vi "Initialize.vi"(2 "error in":errorcluster, 3 "VISA arduino in":refnum<visa-resource-name>) -> (0 "error out":errorcluster, 1 "VISA arduino out":refnum<visa-resource-name>)   [LabVIEW 2021]
uses:
  <vilib>/Instr/_visa.llb/VISA Configure Serial Port (Instr).vi
  <vilib>/Utility/error.llb/Error Cluster From Error Code.vi
  <vilib>/ErrorRing/Error Ring.xnode
panel:
  out "read buffer":string
  out "delay":u32
  out "max iterator":u8
  # "Private"
  # "Public"
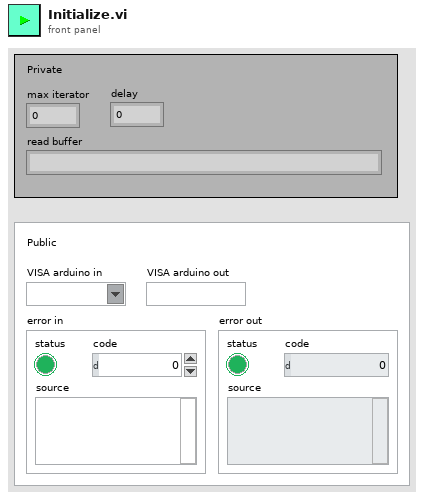
[diagram p1: front panel]
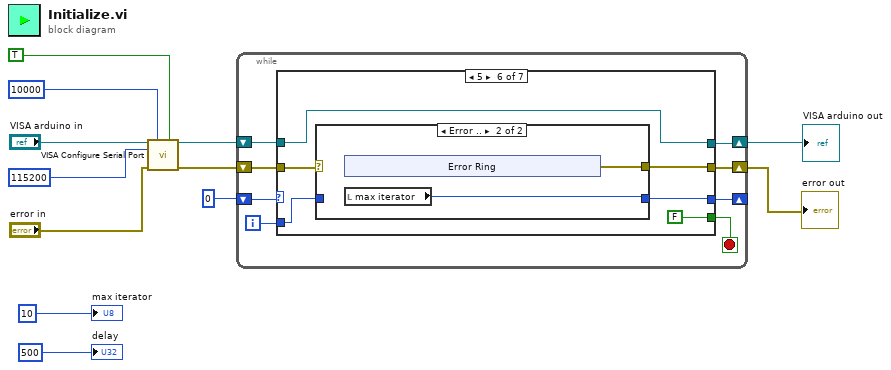
[diagram p0: block diagram]
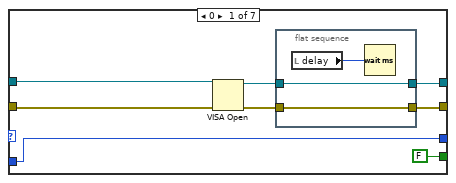
[diagram p2: hidden frame]
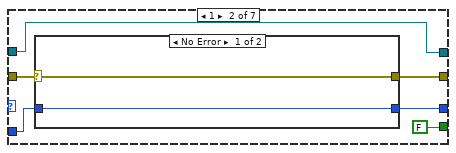
[diagram p3: hidden frame]
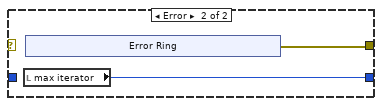
[diagram p4: hidden frame]
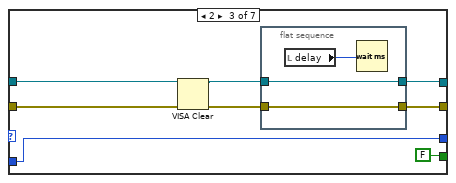
[diagram p5: hidden frame]
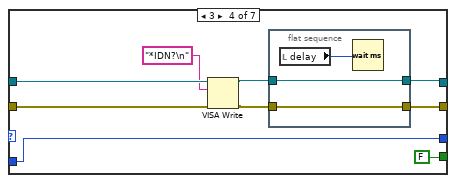
[diagram p6: hidden frame]
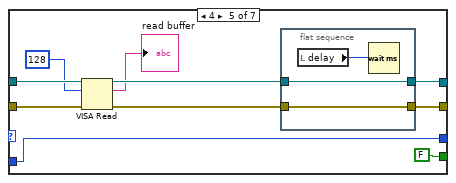
[diagram p7: hidden frame]
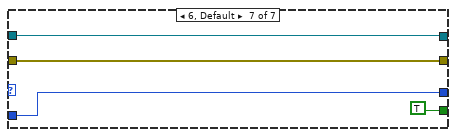
[diagram p9: hidden frame]
diagram:
  n1 = call-poly "VISA Configure Serial Port"("VISA resource name"="VISA arduino in", "timeout (10sec)"=u32 10000, "Enable Termination\nChar (T)"=TRUE ("Enable Termination\nChar (T)"), "baud rate (9600)"=u32 115200, "error in (no error)"="error in") -> ("VISA resource name out"=w9:refnum<visa-resource-name>, "error out"=w8:errorcluster)  [unwired: 9 in]
  n2 = while {
    shift-right: [w18] -> w1
    shift-left: w9 -> [w20]
    shift-right: [w17] -> w2
    shift-left: w8 -> [w19]
    shift-right: [w14] -> _
    shift-left: 0 -> [w16]
    i -> [w15]
    stop <- w13 stop-if-true
    n3 = case shown="5" w16 {
      tunnel: w20 -> [w28 w35 w54 w66 w79 w85 w101]
      tunnel: w19 -> [w27 w37 w53 w65 w78 w87 w100]
      tunnel: [w24 w35 w50 w59 w74 w85 w101] -> w18
      tunnel: [w22 w36 w48 w61 w72 w86 w100] -> w17
      tunnel: w15 -> [w26 w33 w52 w63 w76 w83 w99]
      tunnel: [w26 w34 w52 w63 w76 w84 w99] -> w14
      tunnel: [FALSE ("Enable Termination\nChar (T)") FALSE ("Enable Termination\nChar (T)") FALSE ("Enable Termination\nChar (T)") FALSE ("Enable Termination\nChar (T)") FALSE ("Enable Termination\nChar (T)") FALSE ("Enable Termination\nChar (T)") TRUE ("Enable Termination\nChar (T)")] -> w13
      frame 0 {
        n4 = VISA Open(error in (no error)=w27, VISA resource name=w28) -> (VISA resource name=w23:refnum<visa-resource-name>, error out=w21:errorcluster)  [unwired: 3 in]
        n5 = flat-sequence {
          tunnel: [w30] -> w24
          tunnel: w23 -> [w30]
          tunnel: [w29] -> w22
          tunnel: w21 -> [w29]
          frame #0 {
            n6 = local read "delay"() -> (w31:u32)
            n7 = Wait (ms)(milliseconds to wait=w31) -> ()  [unwired: 1 out]
          }
        }
      }
      frame 1 {
        n8 = case shown="No Error" w37 {
          selector: w37 -> [w39 _]
          tunnel: [w39 w40] -> w36
          tunnel: [w38 w41] -> w34
          tunnel: w33 -> [w38 _]
          frame No Error {
          }
          frame Error {
            n9 = local read "max iterator"() -> (w41:u8)
            n10 = xnode "Error Ring"() -> ("error out"=w40:errorcluster)
          }
        }
      }
      frame 2 {
        n11 = VISA Clear(VISA resource name=w54, error in (no error)=w53) -> (VISA resource name out=w49:refnum<visa-resource-name>, error out=w47:errorcluster)
        n12 = flat-sequence {
          tunnel: [w56] -> w50
          tunnel: w49 -> [w56]
          tunnel: [w55] -> w48
          tunnel: w47 -> [w55]
          frame #0 {
            n13 = local read "delay"() -> (w57:u32)
            n14 = Wait (ms)(milliseconds to wait=w57) -> ()  [unwired: 1 out]
          }
        }
      }
      frame 3 {
        n15 = VISA Write(VISA resource name=w66, write buffer="*IDN?\n", error in (no error)=w65) -> (VISA resource name out=w58:refnum<visa-resource-name>, error out=w60:errorcluster)  [unwired: 1 out]
        n16 = flat-sequence {
          tunnel: [w68] -> w61
          tunnel: w60 -> [w68]
          tunnel: [w67] -> w59
          tunnel: w58 -> [w67]
          frame #0 {
            n17 = local read "delay"() -> (w69:u32)
            n18 = Wait (ms)(milliseconds to wait=w69) -> ()  [unwired: 1 out]
          }
        }
      }
      frame 4 {
        n19 = VISA Read(VISA resource name=w79, byte count=u32 128, error in (no error)=w78) -> (VISA resource name out=w73:refnum<visa-resource-name>, read buffer=→"read buffer":string, error out=w71:errorcluster)  [unwired: 1 out]
        n20 = flat-sequence {
          tunnel: [w81] -> w74
          tunnel: w73 -> [w81]
          tunnel: [w80] -> w72
          tunnel: w71 -> [w80]
          frame #0 {
            n21 = local read "delay"() -> (w82:u32)
            n22 = Wait (ms)(milliseconds to wait=w82) -> ()  [unwired: 1 out]
          }
        }
      }
      frame 5 {
        n23 = case shown="Error .." w87 {
          selector: w87 -> [w90 _]
          tunnel: [w90 w92] -> w86
          tunnel: [w89 w91] -> w84
          tunnel: w83 -> [w89 _]
          frame No Error {
          }
          frame Error {
            n24 = xnode "Error Ring"() -> ("error out"=w92:errorcluster)
            n25 = local read "max iterator"() -> (w91:u8)
          }
        }
      }
      frame 6, Default {
      }
    }
  }
  "VISA arduino out" <- w1
  "error out" <- w2
  "max iterator" <- u8 10 ("Numeric")
  "delay" <- u32 500
